vi "fgv_AO_wave-config.vi"(7 "cmd":T2, 8 "error in (no error)":errorcluster, 11 "Square Wave":T1) -> (0 "error out":errorcluster, 3 "Square Wave 2":T1)   [LabVIEW 2019]
uses:
  _ctrl/rw.ctl
  Set_AO_Wave-config.ctl
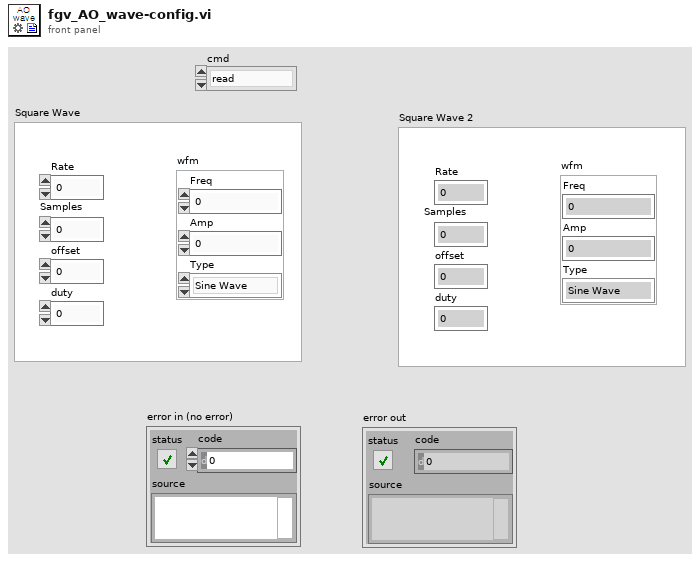
[diagram p1: front panel]
types:
  T1 = typedef "Set_AO_Wave-config.ctl" = cluster{"offset":dbl, "Samples":i32, "duty":dbl, "Rate":dbl, "wfm":cluster{"Freq":dbl, "Amp":dbl, "Type":enum16{"Sine Wave", "Triangle Wave", "Square Wave", "Sawtooth Wave"}}}
  T2 = typedef "rw.ctl" = enum16{"read", "write"}
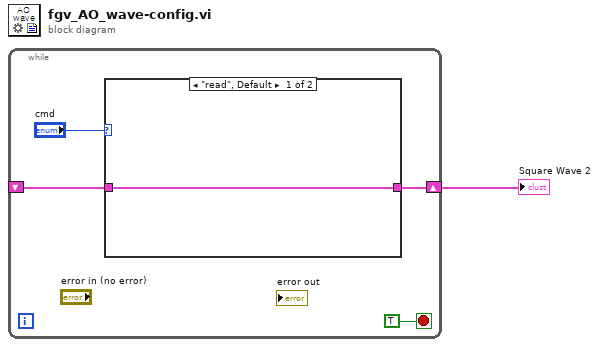
[diagram p0: block diagram]
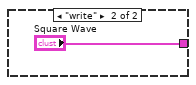
[diagram p2: hidden frame]
diagram:
  n1 = while {
    shift-right: [w3] -> w1
    shift-left: _ -> [w2]
    stop <- TRUE stop-if-true
    n2 = case shown="\"read\", Default" "cmd" {
      tunnel: [w6 "Square Wave"] -> w3
      tunnel: w2 -> [w6 _]
      frame "read", Default {
      }
      frame "write" {
      }
    }
  }
  "Square Wave 2" <- w1
